vi "ThingWorxLabVIEW.vi"(0 "End Session":bool, 3 "Cont Changing Properties":string[][](array[string])=[["Button", "0"], ["Button2", "0"], ["description", ""], ["isConnected", "false"], ["lastConnection", "1970-01-01T00:00:00.000Z"], ["name", "GenericEdge"], ["Photocell", "200"], ["Potentiometer", "234.0"], ["tags", "GenericRemoteEdge:Example"], ["Temperature", "24.2"], ["thingTemplate", "GenericThingTemplate"]], 4 "Select Property to Change":u16(ring)=3 items=["Button", "Button2", "description", "isConnected", "lastConnection", "name", "Photocell", "Potentiometer", "tags", "Temperature", "thingTemplate"], 6 "Desired Value of Property":string="true", 7 "Continuous?":bool=TRUE, 9 "Properties":string[](array[string])=["Button", "Button2", "Photocell", "Potentiometer", "Temperature"], 11 "Input Info":T1={"ThingWorx Server Address"="52.202.159.58", "Port"="80", "Thing Name"="GenericEdge", "Application Key"="0aae8b5f-871a-4973-bdf2-199fabb27dcb", "Service Name"="UpdateValues"}) -> (1 "Properties from ThingWorx":string[][](array[string])=[["Button", "false"], ["Button2", "false"], ["description", ""], ["isConnected", "false"], ["lastConnection", "1970-01-01T00:00:00.000Z"], ["name", "GenericEdge"], ["Photocell", "200.0"], ["Potentiometer", "234.0"], ["tags", "GenericRemoteEdge:Example"], ["Temperature", "2.42"], ["thingTemplate", "GenericThingTemplate"]])   [LabVIEW 2015]
uses:
  Z:/VM Share/ThingWorxLV Summer Work/Sub VIs/SetServiceArrayInputs.vi
panel:
  out "error out":errorcluster
  # "Before running program, input values for \"Thing Name,\" \"App Key,\" \"ThingWorx Server Address,\" \"Port,\"Service Name,\" and \"Properties in Service.\"\nTo change the values of all properties at once, click continuous. If you would like to change individual property values, unclick the continuous\nbutton and select the property you would like to change in the dropdown menu and enter your desired value."
  # "* for booleans, input 0 or 1 for false or true respectively"
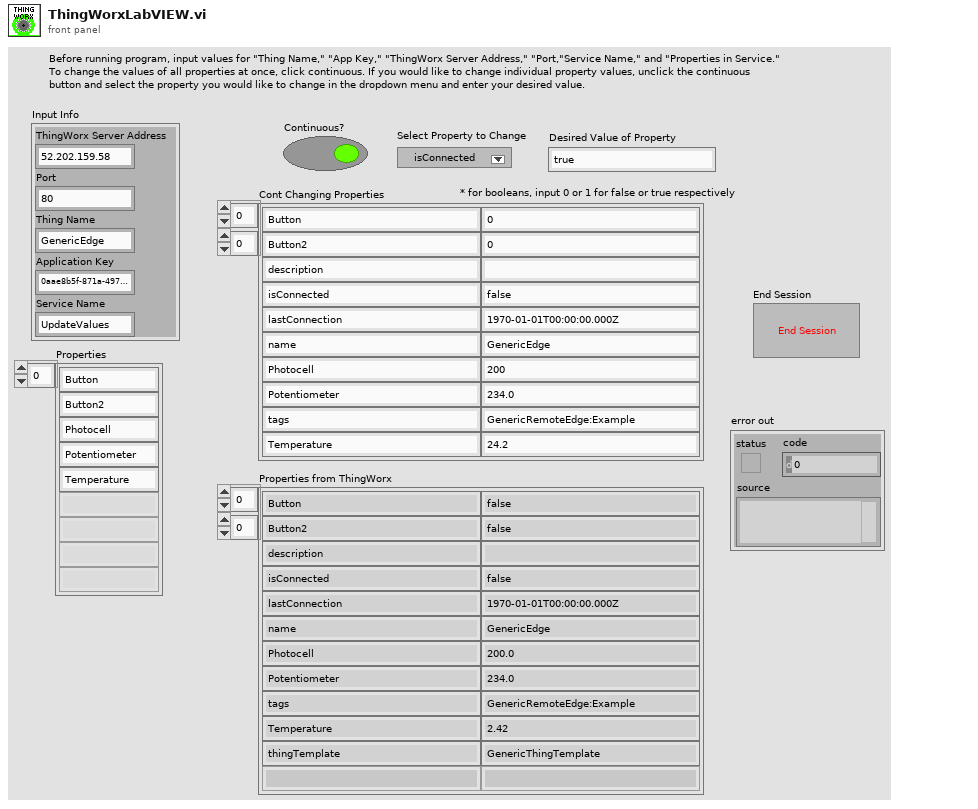
[diagram p1: front panel]
types:
  T1 = cluster{"ThingWorx Server Address":string, "Port":string, "Thing Name":string, "Application Key":string, "Service Name":string}
  T2 = typedef "LabVIEWHTTPClient.lvlib/ClientHandle.ctl" = refnum<k1>
  T3 = cluster{"client handle":T2, "Url Beginning":string, "App Key":string, "Service Name":string, "Properties":string[]}
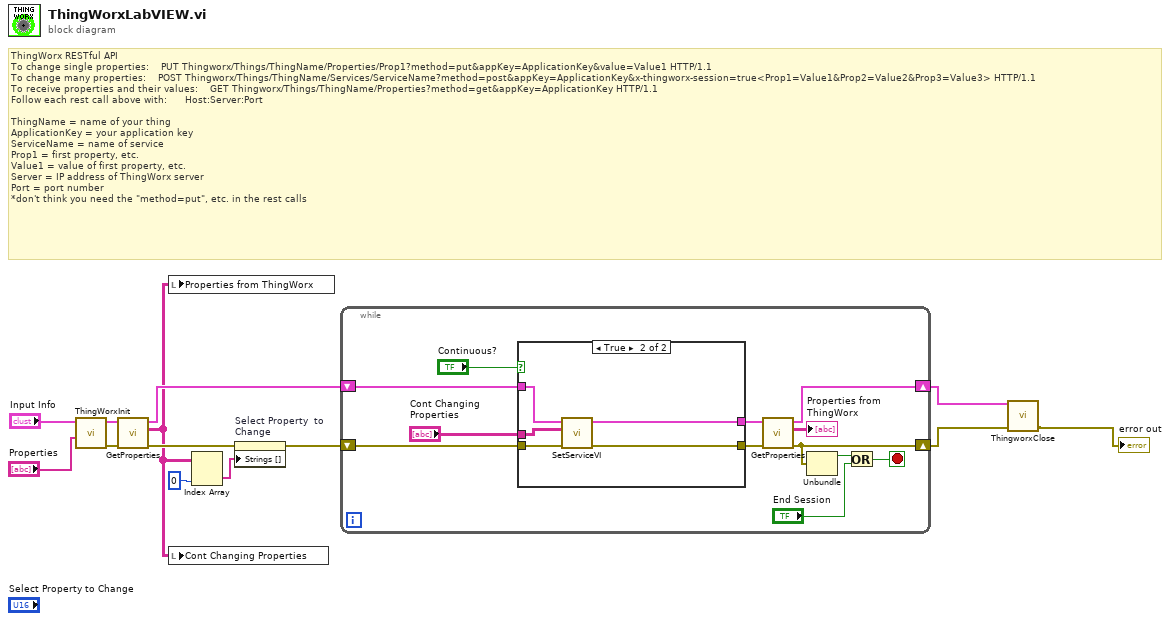
[diagram p0: block diagram]
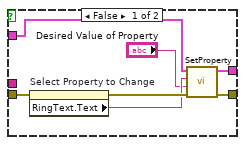
[diagram p2: hidden frame]
diagram:
  # "ThingWorx RESTful API\nTo change single properties:    PUT Thingworx/Things/ThingName/Properties/Prop1?method=put&appKey=ApplicationKey&value=Value1 HTTP/1.1\nTo change many properties:    POST Thingworx/Things/ThingName/Services/ServiceName?method=post&appKey=ApplicationKey&x-thingworx-session=true<Prop1=Value1&Prop2=Value2&Prop3=Value3> HTTP/1.1\nTo receive properties and their values:    GET Thingworx/Things/ThingName/Properties?method=get&appKey=ApplicationKey HTTP/1.1\nFollow each rest call above with:      Host:Server:Port\n\nThingName = name of your thing\nApplicationKey = your application key\nServiceName = name of service\nProp1 = first property, etc.\nValue1 = value of first property, etc.\nServer = IP address of ThingWorx server\nPort = port number\n*don't think you need the \"method=put\", etc. in the rest calls"
  n1 = call "ThingWorxInit.vi"("Properties"="Properties", "Input Info"="Input Info") -> ("error out"=w4:errorcluster, "Thing Info Out"=w5:T3)  [unwired: 8 in]
  n2 = call "GetProperties.vi"("error in (no error)"=w4, "Thing Info In"=w5) -> ("error out"=w9:errorcluster, "Array"=w7:string[][], "Thing Info Out"=w12:T3)  [unwired: 7 in]
  n3 = local write "Properties from ThingWorx"(w7) -> ()
  n4 = local write "Cont Changing Properties"(w7) -> ()
  n5 = Index Array(array=w7, index (col)=0 ("disabled index (col)")) -> (element=w10:string[])  [unwired: 1 in]
  n6 = property on="Select Property  to Change" class="Ring (strict)"(error in=w9, "Strings []"=w10) -> (error out=w8:errorcluster)  [unwired: 1 in, 1 out]
  n7 = while {
    shift-right: [w25] -> w3
    shift-left: w12 -> [w20]
    shift-right: [w16] -> w2
    shift-left: w8 -> [w19]
    stop <- w24 stop-if-true
    n8 = case shown="True" "Continuous?" {
      tunnel: w20 -> [w29 w36]
      tunnel: w19 -> [w31 w34]
      tunnel: [w32 w37] -> w17
      tunnel: [w28 w35] -> w15
      tunnel: "Cont Changing Properties" -> [_ w33]
      frame False {
        n9 = property on="Select Property to Change" class="Ring (strict)"(error in=w31) -> (error out=w30:errorcluster, "RingText.Text"=w27:string)  [unwired: 1 in, 1 out]
        n10 = call "SetProperty.vi"("error in (no error)"=w30, "Value of Property"="Desired Value of Property", "Property"=w27, "Thing Info In"=w29) -> ("error out"=w32:errorcluster, "Thing Info Out"=w28:T3)  [unwired: 6 in]
      }
      frame True {
        n11 = call-poly "SetServiceVI.vi"("error in"=w34, "Properties"=w33, "Thing Info In"=w36) -> ("error out"=w37:errorcluster, "Thing Info Out"=w35:T3)  [unwired: 7 in]
      }
    }
    n12 = call "GetProperties.vi"("error in (no error)"=w17, "Thing Info In"=w15) -> ("error out"=w16:errorcluster, "Array"=→"Properties from ThingWorx":string[][], "Thing Info Out"=w25:T3)  [unwired: 7 in]
    n13 = Unbundle(w16) -> ("status"=w22:bool)  [unwired: 2 out]
    n14 = Or(x=w22, y="End Session") -> (x .or. y?=w24:bool)
  }
  n15 = call "ThingworxClose.vi"("error in (no error)"=w2, "Thing Info Out"=w3) -> ("error out"=→"error out":errorcluster)  [unwired: 3 in]
